vi "3.2.1-VectorNav Write.vi"(9 "Command":string="$VNRRG,08*7B", 10 "error in":errorcluster, 11 "FPGA Ref In":T1) -> (2 "error out":errorcluster, 3 "FPGA VI Reference Out":T1)   [LabVIEW 2010]
doc: "This VI simply takes in a command string, adds a newline character, converts the string to a byte array, and writes this to a DMA FIFO."
uses:
  2-Low Neurons/2-FPGA VI Typedef.ctl
  <vilib>/rvi/interface/nirviMethod/nirviMethod.xnode
  FPGA Bitfiles/DaveBrain_FPGATarget_1-Hindbrain_F0E489D8.lvbitx
  1-Hindbrain.vi
  <vilib>/rvi/interface/common/niFpgaNodeNameForErrorReporting.ctl
  <vilib>/rvi/errors/niLvFpgaWhatHappensToTopLevelVI.ctl
  <vilib>/Utility/error.llb/Error Cluster From Error Code.vi
  <vilib>/rvi/errors/niLvFpgaAdjustHostInterfaceError.vi
  NiFpgaLv.dll
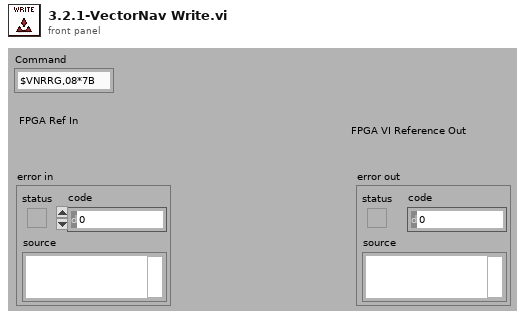
[diagram p1: front panel]
types:
  T1 = typedef "2-FPGA VI Typedef.ctl" = refnum<k20>
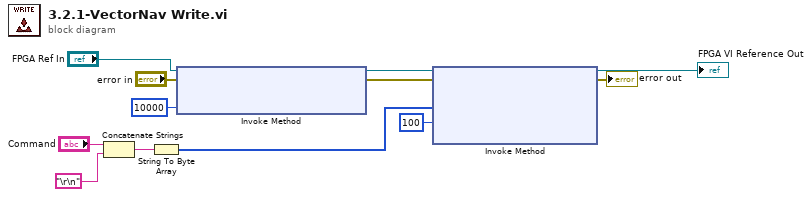
[diagram p0: block diagram]
diagram:
  n1 = Concatenate Strings("Command", "\r\n") -> (w6:string)
  n2 = String To Byte Array(string=w6) -> (unsigned byte array=w9:u8[])
  n3 = xnode "Invoke Method"("FPGA VI Reference In"="FPGA Ref In", "error in"="error in", "Depth"=u32 10000) -> ("FPGA VI Reference Out"=w11:T1, "error out"=w10:errorcluster)
  n4 = xnode "Invoke Method"("FPGA VI Reference In"=w11, "error in"=w10, "Data"=w9, "Timeout (ms)"=100) -> ("FPGA VI Reference Out"=→"FPGA VI Reference Out":T1, "error out"=→"error out":errorcluster)  [unwired: 1 out]
